vi "Read TDMS Props.vi"(0 "DAC in":refnum<class "DAC.lvclass">) -> (4 "DAC out":refnum<class "DAC.lvclass">, 6 "Result Unit":string, 8 "DAC Device":string, 10 "DAC IO":string, 15 "DAC Description":string="Default")   [LabVIEW 2019, in "DAC.lvlib" / "DAC.lvclass"]
uses:
  DAC.lvclass
  DAC.lvclass/DAC.ctl
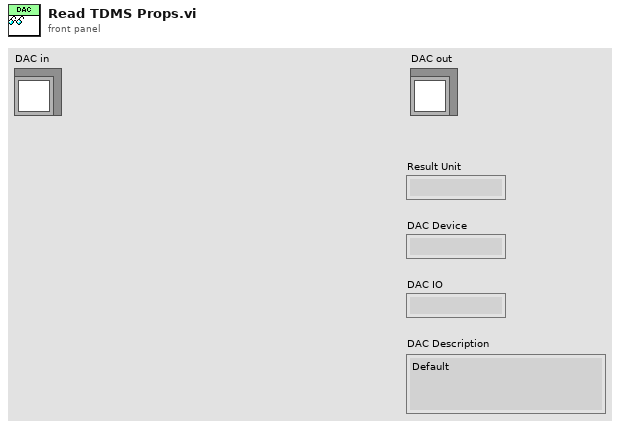
[diagram p1: front panel]
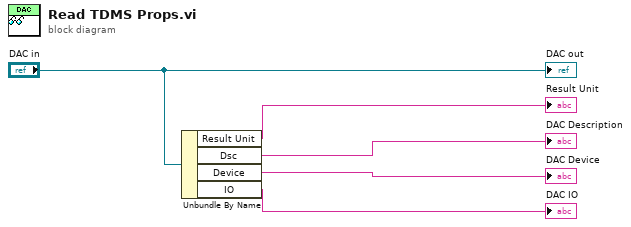
[diagram p0: block diagram]
diagram:
  n1 = Unbundle By Name("DAC in") -> ("Result Unit"=→"Result Unit":string, "Dsc"=→"DAC Description":string, "Device"=→"DAC Device":string, "IO"=→"DAC IO":string)
  "DAC out" <- "DAC in"
